vi "Match Image.vi"(8 "picture":picture, 9 "Template":bool[][](array[boolean]), 11 "rect":T1) -> (3 "%":dbl)   [LabVIEW 2013]
panel:
  out "size(s) 2":i32[](array[numeric])
  out "size(s)":i32[](array[numeric])
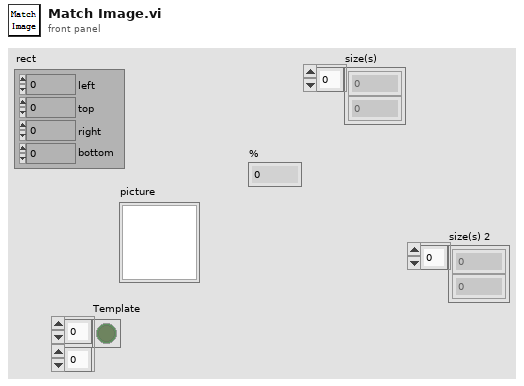
[diagram p1: front panel]
types:
  T1 = cluster{"left":i16, "top":i16, "right":i16, "bottom":i16}
  T2 = typedef "imagedata.ctl" = cluster{"image type":i32, "image depth":i32, "image":u8[], "mask":u8[], "colors":u32[], "Rectangle":cluster{"left":i16, "top":i16, "right":i16, "bottom":i16}}
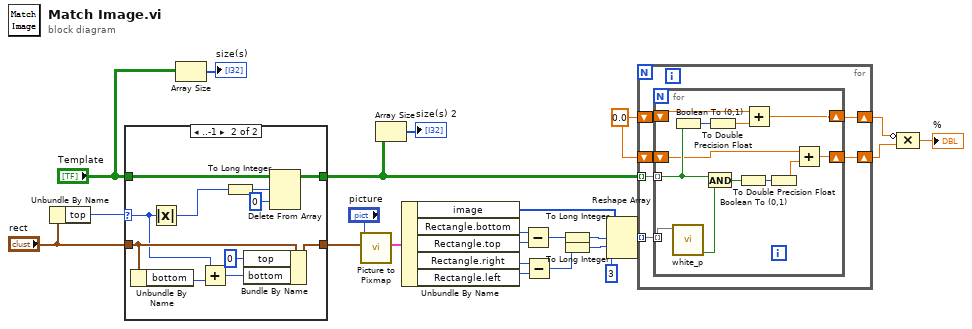
[diagram p0: block diagram]
diagram:
  w8 = 0.0
  n1 = Unbundle By Name("rect") -> ("top"=w9:i16)
  n2 = case shown="..-1" w9 {
    selector: w9 -> [_ w27]
    tunnel: "rect" -> [w26 w30]
    tunnel: [w26 w36] -> w10
    tunnel: "Template" -> [w25 w35]
    tunnel: [w25 w33] -> w1
    frame 0.. {
    }
    frame ..-1 {
      n3 = Unbundle By Name(w30) -> ("bottom"=w29:i16)
      n4 = Absolute Value(x=w27) -> (abs(x)=w34:i16)
      n5 = Add(x=w27, y=w29) -> (x+y=w28:i16)
      n6 = To Long Integer(number=w34) -> (32bit integer=w32:i32)
      n7 = Bundle By Name(cluster=w30, "top"=i16 0, "bottom"=w28) -> (w36:T1)
      n8 = Delete From Array(array=w35, length=w32, index (row)=0) -> (array with subset deleted=w33:bool[][])  [unwired: 1 in, 1 out]
    }
  }
  n9 = Array Size(array="Template") -> (size(s)=→"size(s)":i32[])
  n10 = call <vilib>:"Picture to Pixmap.vi"("rect"=w10, "picture"="picture") -> ("image data"=w19:T2)  [unwired: 8 in, 1 out]
  n11 = Array Size(array=w1) -> (size(s)=→"size(s) 2":i32[])
  n12 = Unbundle By Name(w19) -> ("image"=w22:u8[], "Rectangle.bottom"=w24:i16, "Rectangle.top"=w18:i16, "Rectangle.right"=w17:i16, "Rectangle.left"=w23:i16)
  n13 = Subtract(x=w24, y=w18) -> (x-y=w16:i16)
  n14 = Subtract(x=w17, y=w23) -> (x-y=w15:i16)
  n15 = To Long Integer(number=w16) -> (32bit integer=w14:i32)
  n16 = To Long Integer(number=w15) -> (32bit integer=w13:i32)
  n17 = Reshape Array(w22, w14, w13, 3 ("dimension size")) -> (w20:u8[][][])
  n18 = for {
    tunnel: w20 -> [w43] mode=indexing
    tunnel: w1 -> [w42] mode=indexing
    shift-right: [w40] -> w6
    shift-left: w8 -> [w41]
    shift-right: [w39] -> w7
    shift-left: w8 -> [w38]
    n19 = for {
      tunnel: w43 -> [w44] mode=indexing
      tunnel: w42 -> [w53] mode=indexing
      shift-right: [w51] -> w40
      shift-left: w41 -> [w46]
      shift-right: [w49] -> w39
      shift-left: w38 -> [w47]
      n20 = Boolean To (0,1)(Boolean=w53) -> (0, 1=w52:i16)
      n21 = call "white_p.vi"("Array"=w44) -> ("White"=w45:bool)  [unwired: 10 in]
      n22 = And(x=w53, y=w45) -> (x .and. y?=w55:bool)
      n23 = To Double Precision Float(number=w52) -> (double precision float=w50:dbl)
      n24 = Boolean To (0,1)(Boolean=w55) -> (0, 1=w54:i16)
      n25 = Add(x=w46, y=w50) -> (x+y=w51:dbl)
      n26 = To Double Precision Float(number=w54) -> (double precision float=w48:dbl)
      n27 = Add(x=w47, y=w48) -> (x+y=w49:dbl)
    }
  }
  n28 = Compound Arithmetic op=MULTIPLY(invert w6, w7) -> (→"%":dbl)
